vi "Transfer Force Offsets.vi"(1 "error in":errorcluster, 2 "LVDT In":dbl[][](array[numeric])) -> (0 "error out":errorcluster)   [LabVIEW 2009]
uses:
  Data Access Objects/Metadata/DAO Actions.ctl
  Global Data/Dataset Transaction Id.ctl
  Global Data/Dataset Source.ctl
  Global Data/Dataset Type.ctl
  Apps/Yes No Button.ctl
  Data Access Objects/Metadata/LBCB Number.ctl
  Control Loop/LBCB_Conversions_Actions.ctl
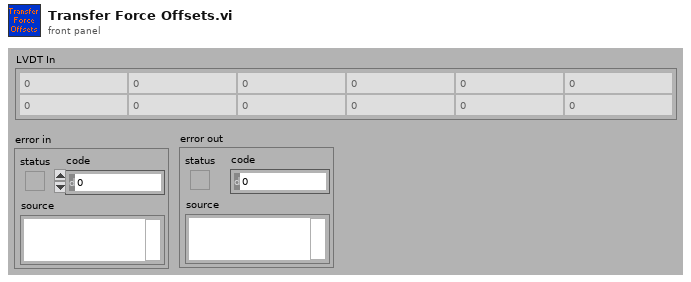
[diagram p1: front panel]
types:
  T1 = typedef "Dataset Type.ctl" = enum16{"LVDT", "Load Cell", "Actuator Command", "Servo Error", "Displacement Command", "Displacement", "Force"}
  T2 = typedef "LBCB Number.ctl" = enum16{"LBCB1", "LBCB2"}
  T3 = typedef "Dataset Source.ctl" = enum16{"LBCB 1", "LBCB 2", "Combined", "External Sensors"}
  T4 = typedef "Dataset Transaction Id.ctl" = cluster{"Dataset Source":T3, "Dataset Type":T1, "Hold":T5, "Volts":T5, "Tag":string}
  T5 = typedef "Yes No Button.ctl" = bool
  T6 = typedef "DAO Actions.ctl" = enum16{"Init", "Get", "Set"}
  T7 = typedef "LBCB Position.ctl" = cluster{"Motion Center":dbl[], "Transformation Matrix":dbl[][]}
  T8 = typedef "LBCB Settings.ctl" = cluster{"Size":T9, "Type":T10}
  T9 = typedef "LBCB Size.ctl" = enum16{"1/5th-scale LBCB", "Full-scale LBCB", "Portable LBCB"}
  T10 = typedef "LBCB Type.ctl" = enum16{"X Actuators On The Left", "X Actuators On The Right"}
  T11 = typedef "LBCB_Conversions_Actions.ctl" = enum16{"A2C", "C2A", "Set Log Filename", "Init"}
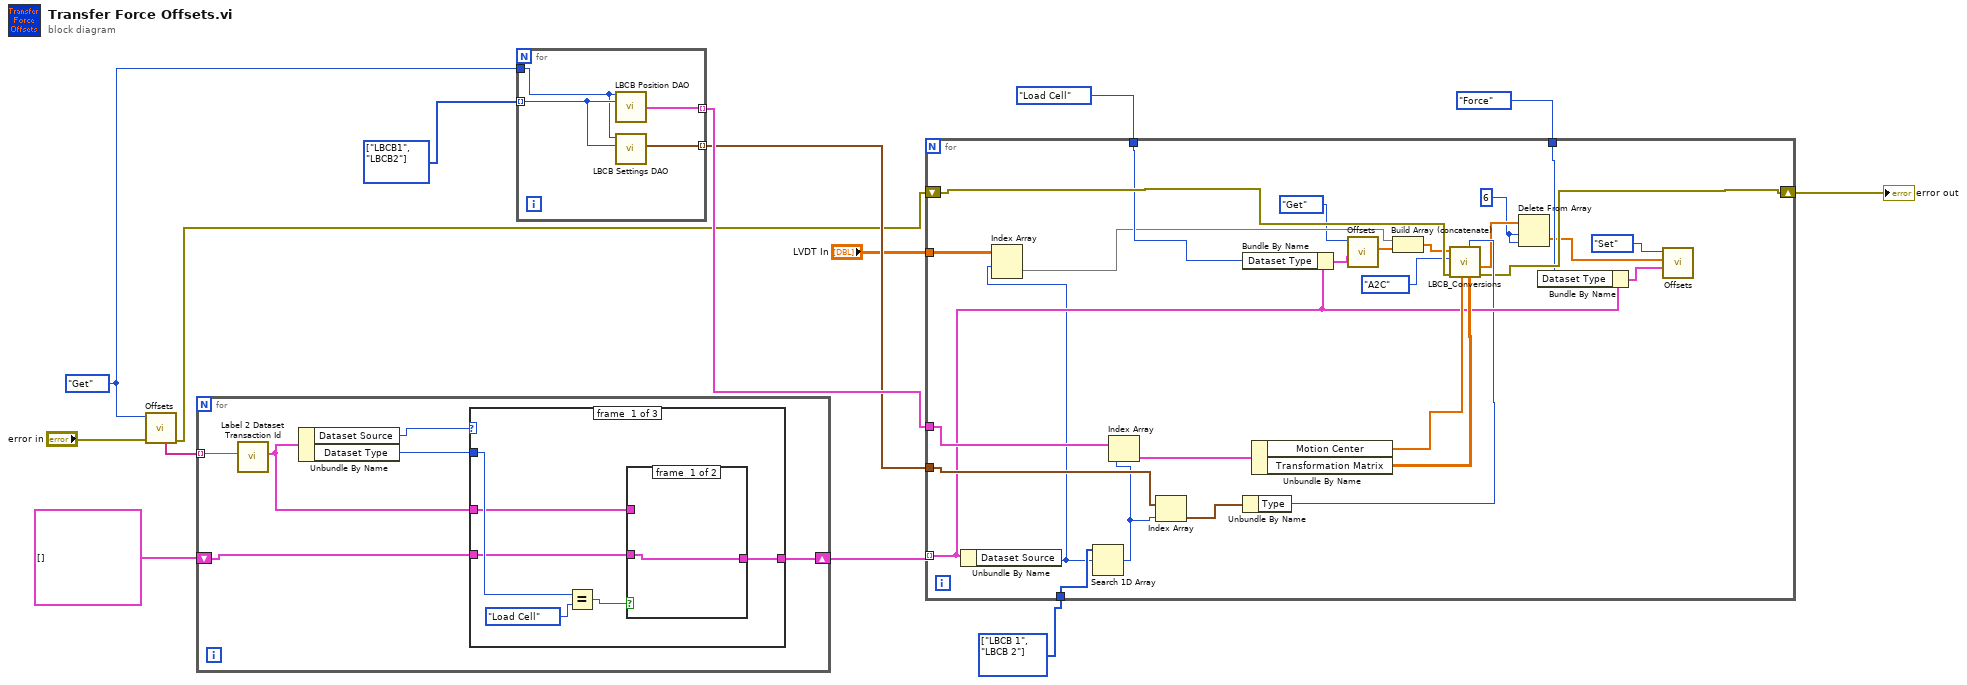
[diagram p0: block diagram]
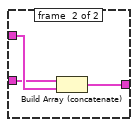
[diagram p2: hidden frame]
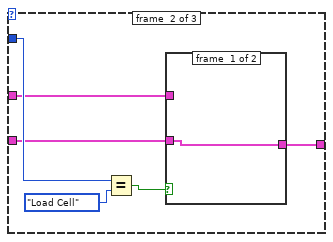
[diagram p3: hidden frame]
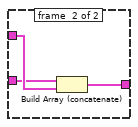
[diagram p4: hidden frame]
diagram:
  w9 = T2[] [enum."LBCB1", enum."LBCB2"] items=["LBCB1", "LBCB2"]
  w11 = T3[] [enum."LBCB 1", enum."LBCB 2"] items=["LBCB 1", "LBCB 2", "Combined", "External Sensors"]
  w8 = DAO_Actions."Get" ("DAO Actions")
  n1 = call "Offsets.vi"("error in (no error)"="error in", "DAO Actions"=w8) -> ("error out"=w5:errorcluster, "Labels"=w13:string[])  [unwired: 7 in, 1 out]
  n2 = for {
    tunnel: w13 -> [w20] mode=indexing
    shift-right: [w16] -> w10
    shift-left: T4[] [] -> [w15]
    n3 = call "Label 2 Dataset Transaction Id.vi"("Label"=w20) -> ("Dataset Trans Id"=w17:T4)  [unwired: 10 in]
    n4 = Unbundle By Name(w17) -> ("Dataset Source"=w19:T3, "Dataset Type"=w18:T1)
    n5 = case shown="\"LBCB 1\"" w19 {
      tunnel: w18 -> [w26 w36 _]
      tunnel: w17 -> [w23 w33 _]
      tunnel: [w22 w32 w41] -> w16
      tunnel: w15 -> [w21 w31 w41]
      frame #0 {
        n6 = Equal?(x=w26, y=Dataset_Type."Load Cell") -> (x = y?=w24:bool)
        n7 = case shown="False" w24 {
          tunnel: w23 -> [_ w30]
          tunnel: [w27 w29] -> w22
          tunnel: w21 -> [w27 w28]
          frame #0 {
          }
          frame #1 {
            n8 = Build Array (concatenate)(w28, w30) -> (w29:T4[])
          }
        }
      }
      frame #1 {
        n9 = Equal?(x=w36, y=Dataset_Type."Load Cell") -> (x = y?=w34:bool)
        n10 = case shown="True" w34 {
          tunnel: w33 -> [_ w40]
          tunnel: [w37 w39] -> w32
          tunnel: w31 -> [w37 w38]
          frame #0 {
          }
          frame #1 {
            n11 = Build Array (concatenate)(w38, w40) -> (w39:T4[])
          }
        }
      }
      frame #2 {
      }
    }
  }
  n12 = for {
    tunnel: w9 -> [w45] mode=indexing
    tunnel: w8 -> [w44]
    tunnel: [w43] -> w7 mode=indexing
    tunnel: [w42] -> w6 mode=indexing
    n13 = call "LBCB Position DAO.vi"("LBCB Settings Actions"=w44, "LBCB Number"=w45) -> ("LBCB Position Output"=w43:T7)  [unwired: 11 in, 2 out]
    n14 = call "LBCB Settings DAO.vi"("LBCB Number"=w45, "Actions"=w44) -> ("LBCB Setting Out"=w42:T8)  [unwired: 7 in, 2 out]
  }
  n15 = for {
    tunnel: w10 -> [w68] mode=indexing
    tunnel: w11 -> [w67]
    tunnel: w7 -> [w72]
    tunnel: w6 -> [w71]
    shift-right: [w61] -> w4
    shift-left: w5 -> [w63]
    tunnel: Dataset_Type."Load Cell" ("Dataset Type") -> [w60]
    tunnel: Dataset_Type."Force" ("Dataset Type") -> [w59]
    tunnel: "LVDT In" -> [w58]
    w47 = 6 ("length")
    n16 = Unbundle By Name(w68) -> ("Dataset Source"=w57:T3)
    n17 = Index Array(array=w58, index (row)=w57) -> (element=w56:dbl[])  [unwired: 1 in]
    n18 = Search 1D Array(1D array=w67, element=w57) -> (index of element=w64:i32)  [unwired: 1 in]
    n19 = Index Array(array=w72, index=w64) -> (element=w66:T7)
    n20 = Index Array(array=w71, index=w64) -> (element=w65:T8)
    n21 = Bundle By Name(cluster=w68, "Dataset Type"=w60) -> (w53:T4)
    n22 = Unbundle By Name(w65) -> ("Type"=w62:T10)
    n23 = Unbundle By Name(w66) -> ("Motion Center"=w70:dbl[], "Transformation Matrix"=w69:dbl[][])
    n24 = call "Offsets.vi"("Dataset Trans Id"=w53, "DAO Actions"=DAO_Actions."Get") -> ("Data Out"=w54:dbl[])  [unwired: 7 in, 2 out]
    n25 = Build Array (concatenate)(w56, w54) -> (w49:dbl[])
    n26 = call "LBCB_Conversions.vi"("Transformation Matrix"=w69, "Type"=w62, "Motion Center"=w70, "error in (no error)"=w63, "Conversion Type"=LBCB_Conversions_Actions."A2C", "Input"=w49) -> ("error out"=w61:errorcluster, "Output"=w50:dbl[])  [unwired: 4 in]
    n27 = Delete From Array(array=w50, length=w47, index=w47) -> (deleted portion=w48:dbl[])  [unwired: 1 out]
    n28 = Bundle By Name(cluster=w68, "Dataset Type"=w59) -> (w52:T4)
    n29 = call "Offsets.vi"("Dataset Trans Id"=w52, "Data In"=w48, "DAO Actions"=DAO_Actions."Set") -> ()  [unwired: 6 in, 3 out]
  }
  "error out" <- w4
